vi "SetEndDate.vi"(8 "error in":errorcluster, 10 "EndDate":timestamp, 11 "StepRun in":refnum<class "StepRun.lvclass">) -> (0 "error out":errorcluster, 3 "StepRun out":refnum<class "StepRun.lvclass">)   [LabVIEW 2021, in "ProligentXMLGenerator.lvlib" / "StepRun.lvclass"]
doc: "Defines the actual date where the step run ended.\n\nThis value is restricted to \"1900-01-01T00:00:00Z\" -\"2100-01-01T00:00:00Z\"."
uses:
  StepRun.lvclass
  StepRun.lvclass/StepRun.ctl
  Base/DateTime/DateTime.lvclass
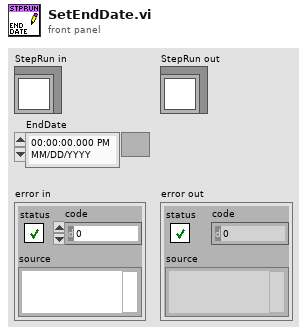
[diagram p1: front panel]
types:
  T1 = typedef "ProligentXMLGenerator.lvlib/StepRun.lvclass/Data.ctl" = cluster{"Name":string, "Measures":refnum<class "Measure.lvclass">[], "FailureReferences":refnum<class "FailureReference.lvclass">[], "Characteristics":refnum<class "Characteristic.lvclass">[], "Documents":refnum<class "Document.lvclass">[], "CustomData":refnum<class "CustomData.lvclass">, "StepExecutionStatus":refnum<class "ExecutionStatus.lvclass">, "StepRunId":refnum<class "Guid.lvclass">, "StepName":refnum<class "NonEmptyString_255.lvclass">, "StartDate":refnum<class "DateTime.lvclass">, "EndDate":refnum<class "DateTime.lvclass">, "TimeZoneInfoId":string}
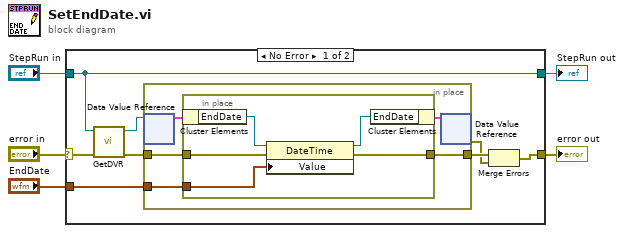
[diagram p0: block diagram]
diagram:
  n1 = case shown="No Error" "error in" {
    selector: "error in" -> [w12 w24]
    tunnel: "StepRun in" -> [w7 w25]
    tunnel: [w9 w24] -> w3
    tunnel: "EndDate" -> [w8 _]
    tunnel: [w7 w25] -> w1
    frame No Error {
      n2 = call "GetDVR.vi"("error in"=w12, "StepRun"=w7) -> ("error out"=w11:errorcluster, "DVRReference"=w13:refnum<data-value>)  [unwired: 8 in]
      n3 = in-place "In Place Element Structure" {
        in-place-border: w11 -> [w16]
        in-place-border: [w18] -> w10
        in-place-border: w8 -> [w17]
        n4 = in-place-dvr #1(w13) -> (w15:T1)  [unwired: 1 out]
        n5 = in-place "In Place Element Structure" {
          in-place-border: [w23] -> w18
          in-place-border: w17 -> [w22]
          in-place-border: w16 -> [w21]
          n6 = in-place-cluster #2(w15) -> ("EndDate"=w20:refnum<class "DateTime.lvclass">)
          n7 = property on="Property Node" class="DateTime"(reference=w20, error in=w21, "Value"=w22) -> (reference out=w19:refnum<class "DateTime.lvclass">, error out=w23:errorcluster)
          n8 = in-place-cluster #2("EndDate"=w19) -> (w14:T1)
        }
        n9 = in-place-dvr #1(w14) -> (w6:errorcluster)  [unwired: 1 out]
      }
      n10 = Merge Errors(w10, w6) -> (w9:errorcluster)
    }
    frame Error {
    }
  }
  "error out" <- w3
  "StepRun out" <- w1
